vi "Choreo_DifferentialSample_Flipped.vi"(11 "ChoreoDifferentialSample":T1={"timestamp"=-999.0, "x"=0.0, "y"=0.0, "heading"=0.0, "velocityL"=0.0, "velocityR"=0.0, "angularVelocity"=0.0, "accelL"=0.0, "accelR"=0.0, "accelAngular"=0.0, "forceL"=0.0, "forceR"=0.0}) -> (3 "FlippedDifferentialSample":T1={"timestamp"=-999.0, "x"=0.0, "y"=0.0, "heading"=0.0, "velocityL"=0.0, "velocityR"=0.0, "angularVelocity"=0.0, "accelL"=0.0, "accelR"=0.0, "accelAngular"=0.0, "forceL"=0.0, "forceR"=0.0})   [LabVIEW 2019, in "ChoreoLib.lvlib"]
doc: "Returns this sample, mirrored across the field midline.\n\nInputs:\n -- ChoreoDifferentialSample - cluster - Differential sample.\n \nOutputs: \n -- FlippedDifferentialSample - cluster - This sample, mirrored across the field midline."
uses:
  ChoreoLib.lvlib
  TypeDef/ChoreoDifferentialSample.ctl
  Choreo_Choreo_Globals.vi
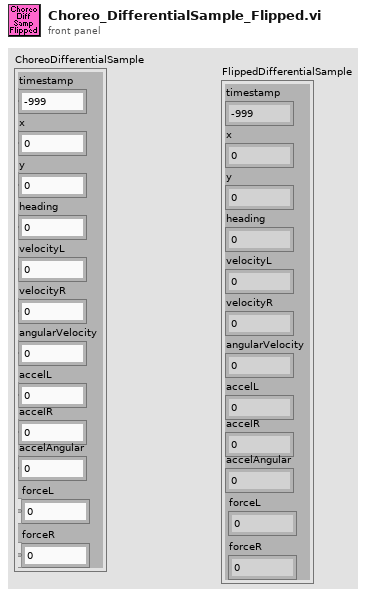
[diagram p1: front panel]
types:
  T1 = typedef "ChoreoLib.lvlib/ChoreoDifferentialSample.ctl" = cluster{"timestamp":dbl, "x":dbl, "y":dbl, "heading":dbl, "velocityL":dbl, "velocityR":dbl, "angularVelocity":dbl, "accelL":dbl, "accelR":dbl, "accelAngular":dbl, "forceL":dbl, "forceR":dbl}
  T2 = typedef "ChoreoLib.lvlib/Choreo_Util_AllianceFlipType.ctl" = enum16{"MIRRORED", "ROTATE_AROUND"}
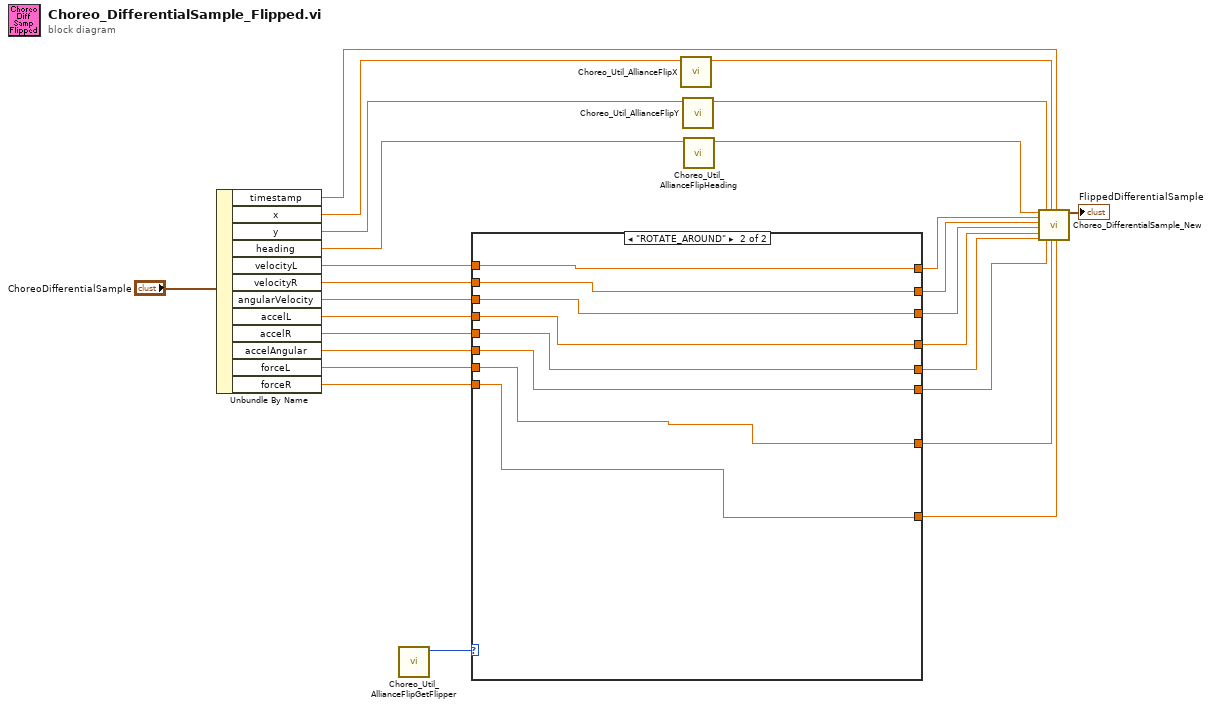
[diagram p0: block diagram]
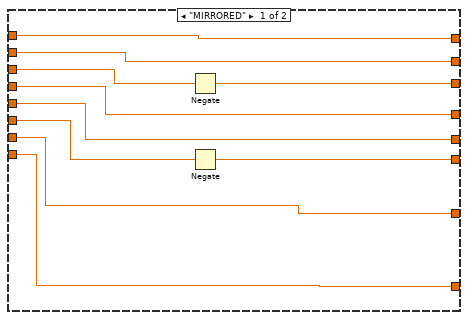
[diagram p2: hidden frame]
diagram:
  n1 = Unbundle By Name("ChoreoDifferentialSample") -> ("timestamp"=w24:dbl, "x"=w21:dbl, "y"=w22:dbl, "heading"=w23:dbl, "velocityL"=w17:dbl, "velocityR"=w16:dbl, "angularVelocity"=w15:dbl, "accelL"=w14:dbl, "accelR"=w13:dbl, "accelAngular"=w12:dbl, "forceL"=w11:dbl, "forceR"=w10:dbl)
  n2 = call "Choreo_Util_AllianceFlipGetFlipper.vi"() -> ("Flipper"=w26:T2)  [unwired: 11 in]
  n3 = case shown="\"ROTATE_AROUND\"" w26 {
    tunnel: w17 -> [w29 w42]
    tunnel: [w36 w41] -> w8
    tunnel: w16 -> [w36 w41]
    tunnel: w15 -> [w35 w44]
    tunnel: w14 -> [w28 w40]
    tunnel: [w34 w39] -> w5
    tunnel: w13 -> [w34 w39]
    tunnel: w12 -> [w33 w43]
    tunnel: w11 -> [w27 w38]
    tunnel: w10 -> [w30 w37]
    tunnel: [w29 w42] -> w9
    tunnel: [w32 w44] -> w7
    tunnel: [w28 w40] -> w6
    tunnel: [w31 w43] -> w4
    tunnel: [w27 w38] -> w3
    tunnel: [w30 w37] -> w2
    frame "MIRRORED" {
      n4 = Negate(x=w35) -> (-x=w32:dbl)
      n5 = Negate(x=w33) -> (-x=w31:dbl)
    }
    frame "ROTATE_AROUND" {
    }
  }
  n6 = call "Choreo_Util_AllianceFlipX.vi"("X"=w21) -> ("FlippedX"=w20:dbl)  [unwired: 10 in]
  n7 = call "Choreo_Util_AllianceFlipY.vi"("Y"=w22) -> ("FlippedY"=w19:dbl)  [unwired: 10 in]
  n8 = call "Choreo_Util_AllianceFlipHeading.vi"("heading"=w23) -> ("FlippedHeading"=w18:dbl)  [unwired: 10 in]
  n9 = call "Choreo_DifferentialSample_New.vi"("heading"=w18, "velocityL"=w9, "velocityR"=w8, "angularVelocity"=w7, "accelL"=w6, "accelR"=w5, "y"=w19, "accelAngular"=w4, "x"=w20, "forceL"=w3, "timestamp"=w24, "forceR"=w2) -> ("ChoreoDifferentialSample"=→"FlippedDifferentialSample":T1)  [unwired: 7 in]
